vi "OAT Find RPM Indices.vi"(7 "reset? (True)":bool=TRUE, 9 "RPM range":cluster{"start":dbl, "end":dbl, "step":dbl} {"step" format="%.2f"; "end" format="%.2f"; "start" format="%.2f"}, 10 "pulse/revolution (1)":i32=1, 11 "speed profile":T1 {"speed [RPM]" format="%.2f"; "time [s]" format="%.2f"}) -> (0 "finished":bool, 1 "RPM scale":cluster{"offset":dbl, "multiplier":dbl} {"multiplier" format="%.2f"; "offset" format="%.2f"}, 2 "time indices":dbl[](array[numeric]) format="%.2f", 3 "rev indices":dbl[](array[numeric]) format="%.2f", 5 "last revolution":dbl format="%.2f")   [LabVIEW 2017]
uses:
  <vilib>/addons/Sound and Vibration/Order Analysis/Tach Process/SubVIs/speed profile.ctl
  <vilib>/addons/Sound and Vibration/Order Analysis/Tach Process/SoundVib_TachProcess.lvlib
panel:
  out "missing":bool
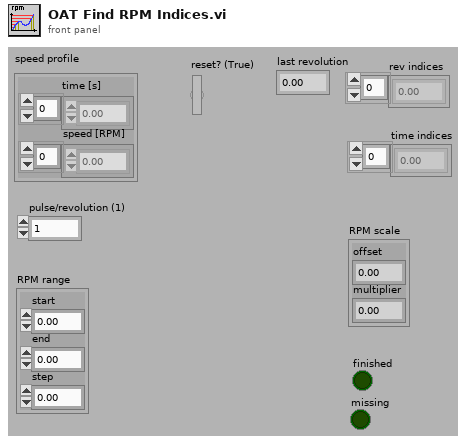
[diagram p1: front panel]
types:
  T1 = typedef "SoundVib_TachProcess.lvlib/speed profile.ctl" = cluster{"time [s]":dbl[], "speed [RPM]":dbl[]}
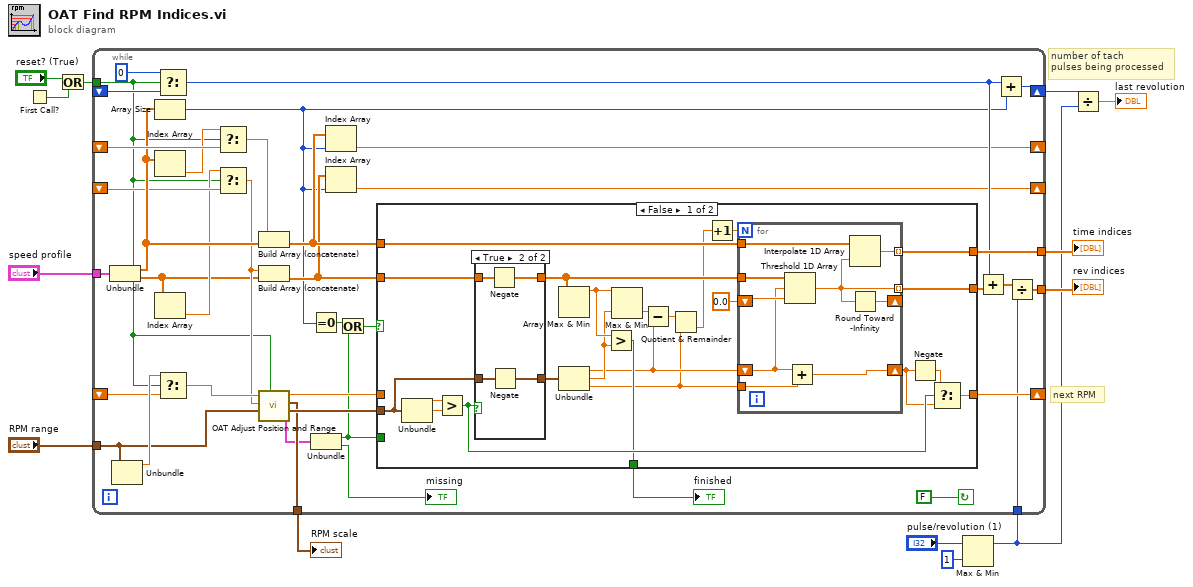
[diagram p0: block diagram]
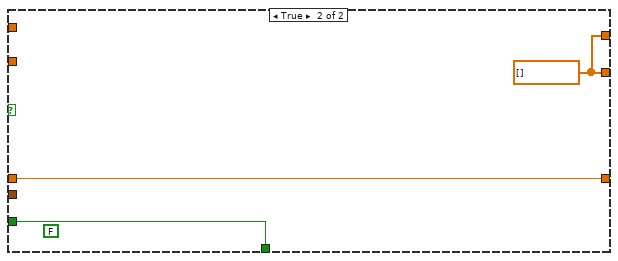
[diagram p3: hidden frame]
diagram:
  # "next RPM"
  # "number of tach\npulses being processed"
  n1 = First Call?() -> (First Call?: T/F=w8:bool)
  n2 = Or(x="reset? (True)", y=w8) -> (x .or. y?=w9:bool)
  n3 = Max & Min(x="pulse/revolution (1)", y=1) -> (max(x,y)=w2:i32)  [unwired: 1 out]
  n4 = while {
    tunnel: "speed profile" -> [w52]
    tunnel: "RPM range" -> [w39]
    tunnel: [w48] -> w7
    tunnel: w9 -> [w14]
    shift-right: [w45] -> w5
    shift-left: _ -> [w47]
    shift-right: [w22] -> _
    shift-left: _ -> [w42]
    tunnel: [w46] -> w11
    tunnel: [w36] -> w6
    shift-right: [w29] -> _
    shift-left: _ -> [w33]
    shift-right: [w23] -> _
    shift-left: _ -> [w31]
    tunnel: w2 -> [w20]
    stop <- FALSE continue-if-true
    n5 = Unbundle(w52) -> ("time [s]"=w32:dbl[], "speed [RPM]"=w19:dbl[])
    n6 = Unbundle(w39) -> ("start"=w43:dbl)  [unwired: 2 out]
    n7 = Array Size(array=w32) -> (size(s)=w18:i32)
    n8 = Index Array(array=w32) -> (element=w27:dbl)  [unwired: 1 in]
    n9 = Index Array(array=w19) -> (element=w26:dbl)  [unwired: 1 in]
    n10 = Select(t=0, s=w14, f=w47) -> (s? t:f=w44:i32)
    n11 = Select(t=w43, s=w14, f=w42) -> (s? t:f=w40:dbl)
    n12 = Select(t=w27, s=w14, f=w33) -> (s? t:f=w28:dbl)
    n13 = Select(t=w26, s=w14, f=w31) -> (s? t:f=w24:dbl)
    n14 = Build Array (concatenate)(w28, w32) -> (w30:dbl[])
    n15 = Build Array (concatenate)(w24, w19) -> (w25:dbl[])
    n16 = call <vilib>:"OAT Adjust Position and Range.vi"("reset"=w14, "range in"=w39, "start position"=w24, "current position"=w40) -> ("flags"=w35:cluster{"finished":bool, "data missed":bool}, "range out"=w38:cluster{"start":dbl, "end":dbl, "step":dbl}, "scale"=w36:cluster{"offset":dbl, "multiplier":dbl}, "current position out"=w37:dbl)  [unwired: 4 in]
    n17 = Equal To 0?(x=w18) -> (x = 0?=w17:bool)
    n18 = Unbundle(w35) -> ("finished"=w15:bool, "data missed"=→"missing":bool)
    n19 = Index Array(array=w30, index=w18) -> (element=w29:dbl)
    n20 = Index Array(array=w25, index=w18) -> (element=w23:dbl)
    n21 = Or(x=w17, y=w15) -> (x .or. y?=w16:bool)
    n22 = case shown="False" w16 {
      tunnel: w38 -> [w66 _]
      tunnel: w25 -> [w73 _]
      tunnel: [w69 w92] -> w22
      tunnel: [w54 w93] -> w50
      tunnel: w30 -> [w70 _]
      tunnel: [w53 w93] -> w46
      tunnel: [w62 w91] -> w21
      tunnel: w37 -> [_ w92]
      tunnel: w15 -> [_ w91]
      frame False {
        n23 = Unbundle(w66) -> ("start"=w75:dbl, "end"=w74:dbl)  [unwired: 1 out]
        n24 = Greater?(x=w75, y=w74) -> (0:w67:bool)
        n25 = case shown="True" w67 {
          tunnel: w73 -> [w86 w90]
          tunnel: w66 -> [w85 w89]
          tunnel: [w86 w88] -> w65
          tunnel: [w85 w87] -> w72
          frame False {
          }
          frame True {
            n26 = Negate(x=w90) -> (-x=w88:dbl[])
            n27 = Negate(x=w89) -> (-x=w87:cluster{"start":dbl, "end":dbl, "step":dbl})
          }
        }
        n28 = Array Max & Min(array=w65) -> (max value=w64:dbl)  [unwired: 3 out]
        n29 = Unbundle(w72) -> ("start"=w60:dbl, "end"=w63:dbl, "step"=w58:dbl)
        n30 = Greater?(x=w64, y=w63) -> (0:w62:bool)
        n31 = Max & Min(x=w64, y=w63) -> (min(x,y)=w61:dbl)  [unwired: 1 out]
        n32 = Subtract(x=w61, y=w60) -> (x-y=w59:dbl)
        n33 = Quotient & Remainder(x=w59, y=w58) -> (floor(x/y)=w57:dbl)  [unwired: 1 out]
        n34 = Increment(x=w57) -> (x+1=w55:dbl)
        n35 = for {
          N: w55 -> [_]
          tunnel: w65 -> [w84]
          shift-right: [w81] -> w56
          shift-left: w60 -> [w80]
          shift-right: [w76] -> _
          shift-left: 0.0 -> [w83]
          tunnel: w58 -> [w82]
          tunnel: [w77] -> w54 mode=indexing
          tunnel: w70 -> [w79]
          tunnel: [w78] -> w53 mode=indexing
          n36 = Threshold 1D Array(1:w83, 2:w80, 3:w84) -> (0:w77:dbl)
          n37 = Add(x=w80, y=w82) -> (x+y=w81:dbl)
          n38 = Interpolate 1D Array(1:w77, 2:w79) -> (0:w78:dbl)
          n39 = Round Toward -Infinity(1:w77) -> (0:w76:dbl)
        }
        n40 = Negate(x=w56) -> (-x=w68:dbl)
        n41 = Select(t=w68, s=w67, f=w56) -> (s? t:f=w69:dbl)
      }
      frame True {
        (unwired) FALSE
        w93 = dbl[] []
      }
    }
    "finished" <- w21
    n42 = Add(x=w44, y=w50) -> (x+y=w49:dbl[])
    n43 = Add(x=w44, y=w18) -> (x+y=w45:i32)
    n44 = Divide(x=w49, y=w20) -> (x/y=w48:dbl[])
  }
  "rev indices" <- w7
  "time indices" <- w11
  "RPM scale" <- w6
  n45 = Divide(x=w5, y=w2) -> (x/y=→"last revolution":dbl)
